vi "Ctor.vi"(8 "error in (no error)":errorcluster, 10 "SQLite":refnum<class "SQLite.lvclass">) -> (0 "error out":errorcluster, 3 "Challenge DB out":refnum<class "Challenge DB.lvclass">)   [LabVIEW 2020, in "Summer of LabVIEW.lvlib" / "Challenge DB.lvclass"]
uses:
  Challenge DB.lvclass
  Challenge DB.lvclass/Challenge DB.ctl
  SQLite/SQLite.lvclass
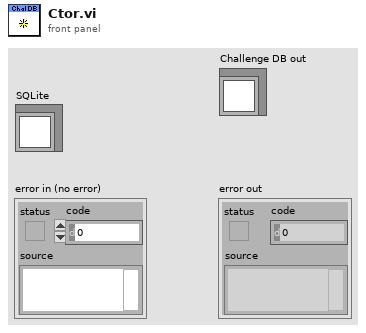
[diagram p1: front panel]
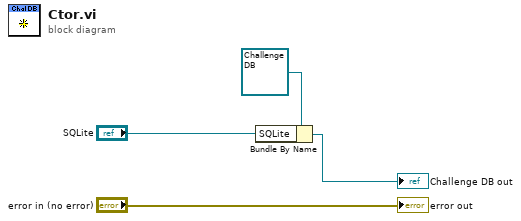
[diagram p0: block diagram]
diagram:
  n1 = Bundle By Name(cluster=refnum<class "Challenge DB.lvclass"> refnum ("Challenge DB in"), "SQLite"="SQLite") -> (→"Challenge DB out":refnum<class "Challenge DB.lvclass">)
  "error out" <- "error in (no error)"
